vi "Offset _fgv.vi"(2 "error in (no error)":errorcluster, 3 "mode":enum16{"read", "write"}(ring), 4 "Value  in":dbl) -> (0 "error out":errorcluster, 1 "Value out":dbl)   [LabVIEW 2019]
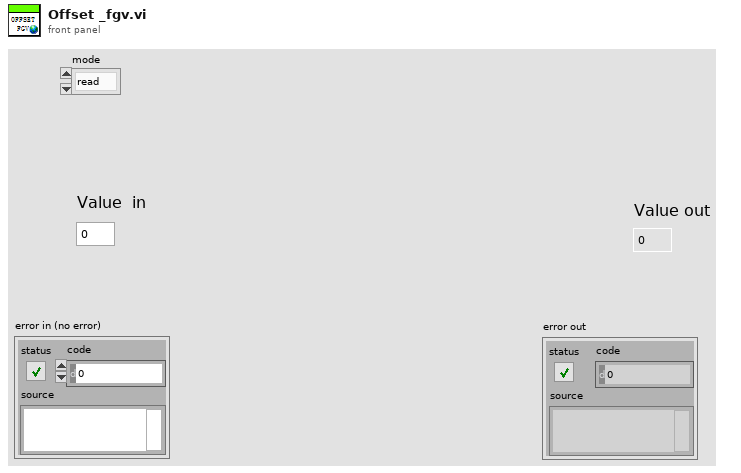
[diagram p1: front panel]
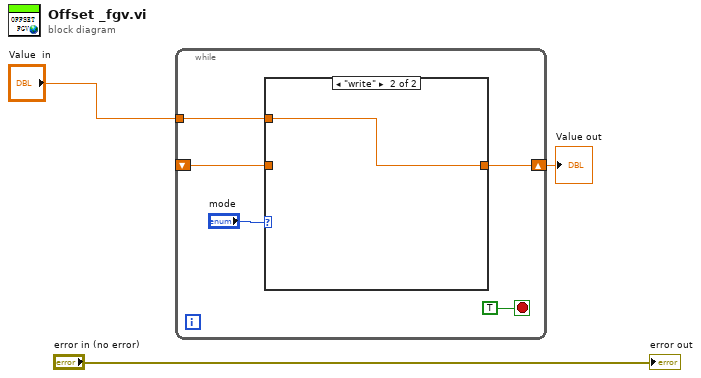
[diagram p0: block diagram]
diagram:
  n1 = while {
    tunnel: "Value  in" -> [w8]
    shift-right: [w7] -> w1
    shift-left: _ -> [w6]
    stop <- TRUE stop-if-true
    n2 = case shown="\"write\"" "mode" {
      tunnel: [w9 w10] -> w7
      tunnel: w8 -> [_ w10]
      tunnel: w6 -> [w9 _]
      frame "read", Default {
      }
      frame "write" {
      }
    }
  }
  "Value out" <- w1
  "error out" <- "error in (no error)"
